vi "Check Device Type.vi"(8 "error in (no error)":errorcluster, 9 "Device Type Name":string, 10 "Ambient Light Bricklet in":refnum<class "Ambient Light Bricklet.lvclass">) -> (0 "error out":errorcluster, 1 "correct Device":bool, 2 "Ambient Light Bricklet out":refnum<class "Ambient Light Bricklet.lvclass">)   [LabVIEW 2011, in "Tinkerforge.lvlib" / "Ambient Light Bricklet.lvclass"]
doc: "This VI is the child implementation of \"Check Device Type.vi\" and invokes the device type validation through checking the device name."
uses:
  Ambient Light Bricklet.lvclass
  Device/Device.lvclass
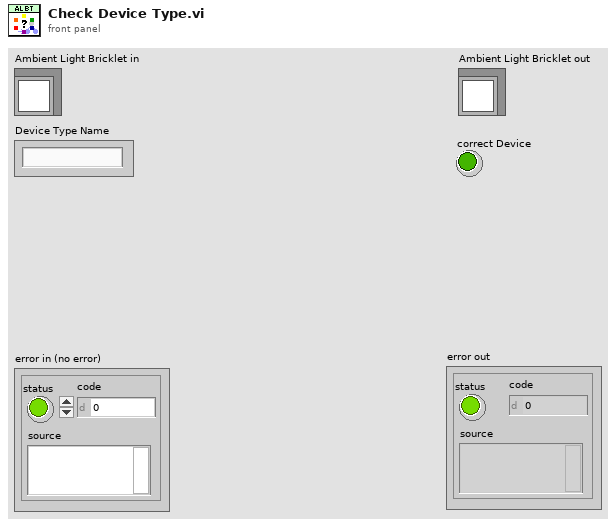
[diagram p1: front panel]
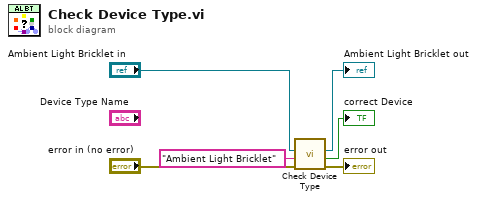
[diagram p0: block diagram]
diagram:
  n1 = call-parent "Check Device Type.vi"("error in (no error)"="error in (no error)", "Device Type Name"="Ambient Light Bricklet", "Device in"="Ambient Light Bricklet in") -> ("error out"=→"error out":errorcluster, "correct Device"=→"correct Device":bool, "Device out"=→"Ambient Light Bricklet out":refnum<class "Ambient Light Bricklet.lvclass">)  [unwired: 6 in]
